vi "init.vi"(8 "error in (no error)":errorcluster, 9 "inputs":u16[][](array[numeric]), 10 "time_stamp":timestamp, 11 "MeasurementResult in":refnum<class "MeasurementDatalvclass.lvclass">) -> (0 "error out":errorcluster, 3 "MeasurementResult out":refnum<class "MeasurementDatalvclass.lvclass">)   [LabVIEW 2017, in "MeasurementDatalvclass.lvclass"]
doc: "Create a new MeasurementResult object"
uses:
  MeasurementDatalvclass.lvclass
  MeasurementDatalvclass.lvclass/MeasurementDatalvclass.ctl
panel:
  # "2d array of u16"
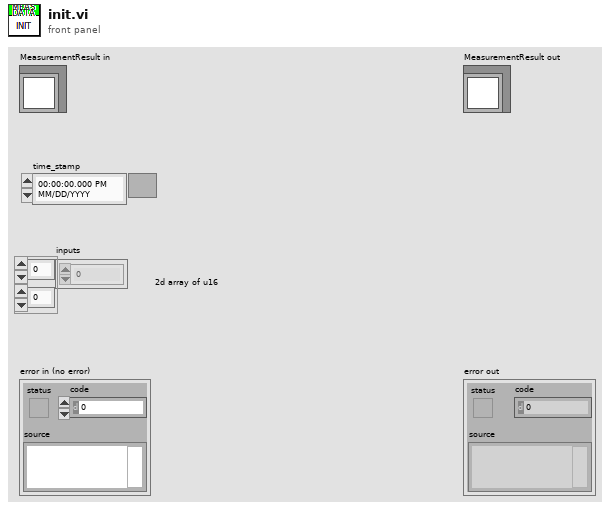
[diagram p1: front panel]
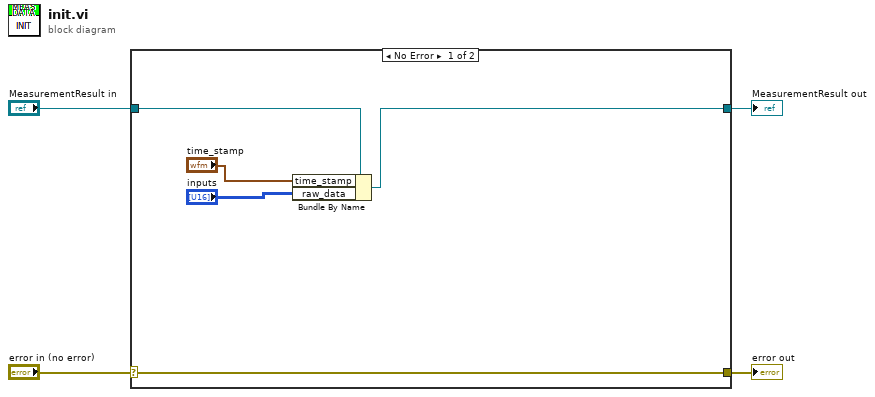
[diagram p0: block diagram]
diagram:
  n1 = case shown="No Error" "error in (no error)" {
    selector: "error in (no error)" -> [w9 w11]
    tunnel: [w9 w11] -> w3
    tunnel: [w7 w10] -> w1
    tunnel: "MeasurementResult in" -> [w8 w10]
    frame No Error {
      n2 = Bundle By Name(cluster=w8, "time_stamp"="time_stamp", "raw_data"="inputs") -> (w7:refnum<class "MeasurementDatalvclass.lvclass">)
    }
    frame Error {
    }
  }
  "error out" <- w3
  "MeasurementResult out" <- w1
